vi "run.vi"(8 "error in (no error)":errorcluster, 11 "S4ICS in":refnum<class "S4ICS.lvclass">) -> (0 "error out":errorcluster, 3 "S4ICS out":refnum<class "S4ICS.lvclass">)   [LabVIEW 2018, in "S4ICS.lvclass"]
uses:
  S4ICS.lvclass
  S4ICS.lvclass/S4ICS.ctl
  State Machine/State Machine.lvclass
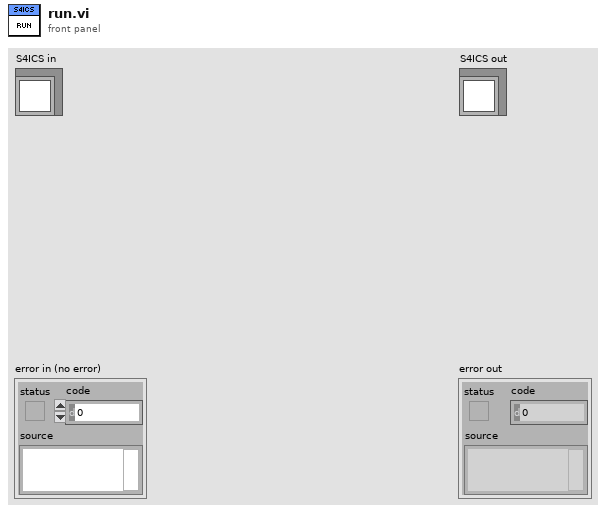
[diagram p1: front panel]
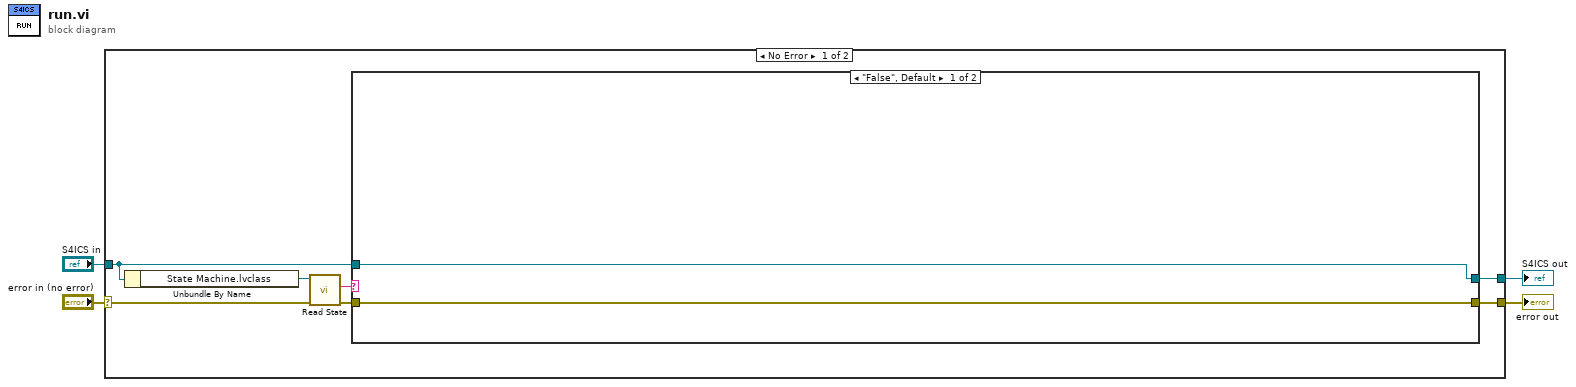
[diagram p0: block diagram]
diagram:
  n1 = case shown="No Error" "error in (no error)" {
    selector: "error in (no error)" -> [w10 w17]
    tunnel: [w5 w17] -> w3
    tunnel: [w7 w16] -> w1
    tunnel: "S4ICS in" -> [w8 w16]
    frame No Error {
      n2 = Unbundle By Name(w8) -> ("State Machine.lvclass"=w11:refnum<class "State Machine.lvclass">)
      n3 = call-dynamic "Read State.vi"("error in (no error)"=w10, "State Machine in"=w11) -> ("error out"=w6:errorcluster, "State"=w9:string)  [unwired: 7 in, 1 out]
      n4 = case shown="\"False\", Default" w9 {
        tunnel: w8 -> [w13 w15]
        tunnel: [w13 w15] -> w7
        tunnel: w6 -> [w12 w14]
        tunnel: [w12 w14] -> w5
        frame "False", Default {
        }
        frame "-----------------" {
        }
      }
    }
    frame Error {
    }
  }
  "error out" <- w3
  "S4ICS out" <- w1
